vi "Arduino_PID_mit 4725_Spannungsregelung.vi"() -> ()   [LabVIEW 2014]
uses:
  <vilib>/MakerHub/LINX/Public/Peripherals/Analog/Analog Read 1 Chan.vi
  <vilib>/MakerHub/LINX/Public/Peripherals/Analog/Analog Read N Chans.vi
  <vilib>/MakerHub/LINX/Private/Local IO/LinxI2cWrite.vi
  <vilib>/MakerHub/LINX/Public/Utilities/Check Channel.vi
  <vilib>/MakerHub/LINX/Private/Local IO/LinxAnalogRead.vi
  <vilib>/MakerHub/LINX/Public/Utilities/Open Serial.vi
  <vilib>/MakerHub/LINX/Private/Utilties/Generate Error.vi
  <vilib>/addons/control/pid/pid.llb/PID (DBL).vi
  <vilib>/MakerHub/LINX/LMH-LINX.lvlib
  <vilib>/addons/control/pid/NI_PID_pid.lvlib
panel:
  out "Device Name":string
  out "Signalverlaufsdiagramm 2":dbl(graph)
  out "Signalverlaufsdiagramm":cluster{"setpoint":dbl, "Voltage":dbl}(graph)
  in  "output range":cluster{"output high":dbl, "output low":dbl}={"output high"=100.0, "output low"=-100.0} caption="Ausgangsbereich" {"output low" format="%.2f"; "output high" format="%.2f"}
  out "output":dbl(knob) caption="Stellgröße x" scale=0.0..10.0
  in  "PID gains":T1={"proportional gain (Kc)"=1.0, "integral time (Ti, min)"=0.01, "derivative time (Td, min)"=0.0} caption="PID-Verstärkungswerte" {"derivative time (Td, min)" format="%.3f"; "integral time (Ti, min)" format="%.3f"; "proportional gain (Kc)" format="%.3f"}
  in  "setpoint":dbl caption="Sollwert" format="%.2f"
  out "Volt":dbl
  in  "Analog Channel":u8
  in  "stop":bool
  in  "Serial Port":refnum<visa-resource-name>="N/A"
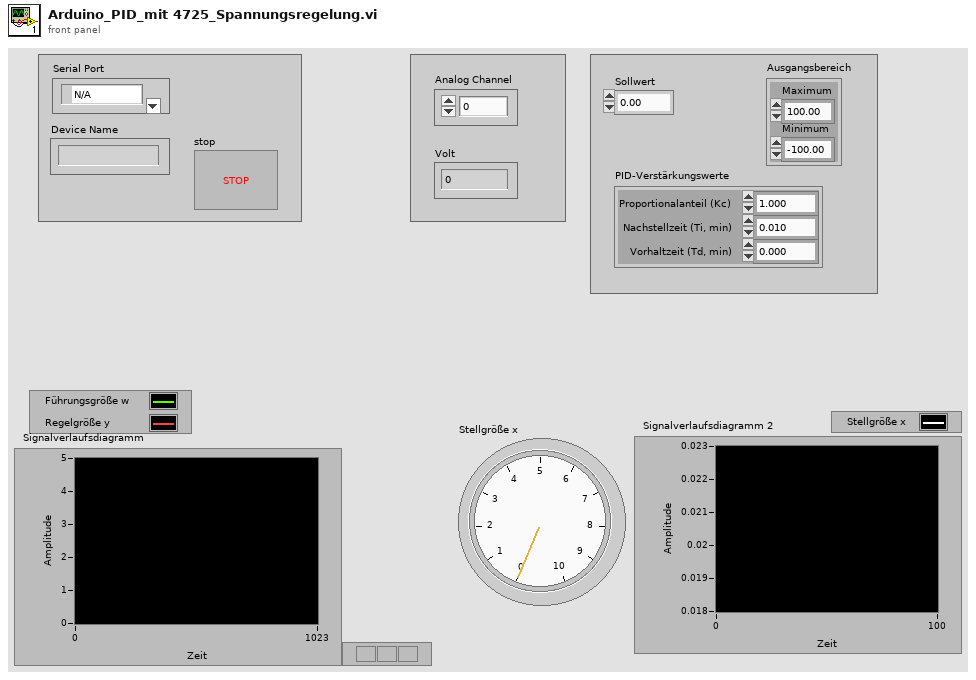
[diagram p1: front panel]
types:
  T1 = cluster{"proportional gain (Kc)":dbl, "integral time (Ti, min)":dbl, "derivative time (Td, min)":dbl}
  T2 = typedef "LMH-LINX.lvlib/LINX Ref.ctl" = cluster{"IO":T3, "Interface":T4, "LINX Device Config":T5}
  T3 = typedef "LMH-LINX.lvlib/Platform.ctl" = enum16{"Remote", "Local"}
  T4 = typedef "LMH-LINX.lvlib/Interface.ctl" = enum16{"Serial", "TCP"}
  T5 = typedef "LMH-LINX.lvlib/Device.lvlib/LINX Device Config.ctl" = cluster{"Interface":T4, "COM Port":refnum<visa-resource-name>, "TCP Configuration":T6, "Device Family":u8, "Device ID":u8, "Device Name":string, "TCP Ref":refnum<k5>, "Channels":T7}
  T6 = typedef "LMH-LINX.lvlib/Device.lvlib/TCP Config.ctl" = cluster{"IP Address":string, "Port":u16}
  T7 = typedef "LMH-LINX.lvlib/Channels.ctl" = cluster{"DI":u8[], "DO":u8[], "AI":u8[], "AO":u8[], "PWM":u8[], "QE":u8[], "UART":u8[], "I2C 2":u8[], "SPI":u8[], "CAN":u8[], "Servo":u8[], "AI Ref (V)":dbl, "AI Resolution (Bits)":u8, "AO Ref (V)":dbl, "AO Resolution (Bits)":u8}
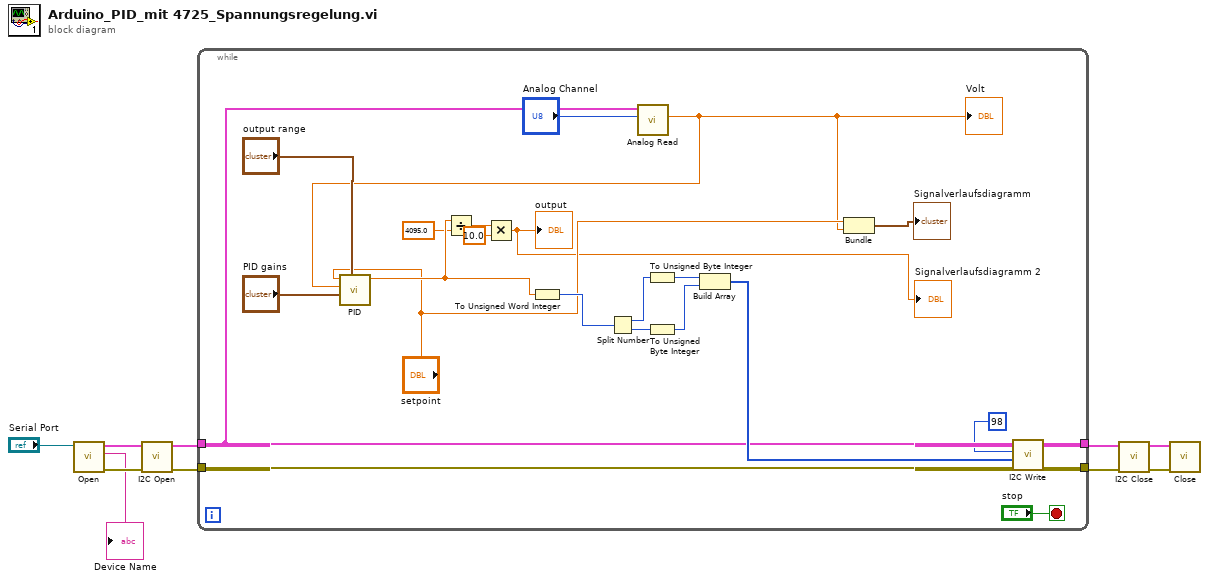
[diagram p0: block diagram]
diagram:
  n1 = call-poly <vilib>:"Open.vi"("Serial Port"="Serial Port") -> ("Error Out"=w10:errorcluster, "Device Name"=→"Device Name":string, "LINX Resource"=w6:T2)  [unwired: 8 in]
  n2 = call <vilib>:"I2C Open.vi"("Error In"=w10, "LINX Resource"=w6) -> ("Error Out"=w7:errorcluster, "LINX Resource"=w8:T2)  [unwired: 8 in]
  n3 = while {
    tunnel: w8 -> [w22]
    tunnel: w7 -> [w29]
    tunnel: [w33] -> w5
    tunnel: [w32] -> w4
    stop <- "stop" stop-if-true
    n4 = call-poly <vilib>:"Analog Read.vi"("Analog Channel"="Analog Channel", "LINX Resource"=w22) -> ("Voltage"=w13:dbl)  [unwired: 6 in, 3 out]
    "Volt" <- w13
    n5 = call-poly <vilib>:"PID.vi"("output range"="output range", "PID gains"="PID gains", "process variable"=w13, "setpoint"="setpoint") -> ("output"=w17:dbl)  [unwired: 6 in, 1 out]
    n6 = Divide(x=w17, y=4095.0) -> (x/y=w18:dbl)
    n7 = Multiply(x=w18, y=10.0) -> (x*y=→"output" →"Signalverlaufsdiagramm 2":dbl)
    n8 = To Unsigned Word Integer(number=w17) -> (unsigned 16bit integer=w23:u16)
    n9 = Split Number(x=w23) -> (hi(x)=w25:u8, lo(x)=w30:u8)
    n10 = To Unsigned Byte Integer(number=w25) -> (unsigned 8bit integer=w26:u8)
    n11 = To Unsigned Byte Integer(number=w30) -> (unsigned 8bit integer=w27:u8)
    n12 = Build Array(w26, w27) -> (w24:u8[])
    n13 = Bundle("setpoint"="setpoint", "Voltage"=w13) -> (→"Signalverlaufsdiagramm":cluster{"setpoint":dbl, "Voltage":dbl})  [unwired: 1 in]
    n14 = call <vilib>:"I2C Write.vi"("Error In"=w29, "Data"=w24, "I2C Slave Address (0)"=u8 98, "LINX Resource"=w22) -> ("Error Out"=w32:errorcluster, "LINX Resource"=w33:T2)  [unwired: 6 in]
  }
  n15 = call <vilib>:"I2C Close.vi"("Error In"=w4, "LINX Resource"=w5) -> ("Error Out"=w3:errorcluster, "LINX Resource"=w2:T2)  [unwired: 8 in]
  n16 = call <vilib>:"Close.vi"("Error In"=w3, "LINX Resource"=w2) -> ()  [unwired: 9 in, 1 out]
